vi "AIM664 Loopback.vi"() -> ()   [LabVIEW 2020]
uses:
  typedefs/BoardControlControl.ctl
  typedefs/BoardControlPortConfig.ctl
  typedefs/BoardControlGoodLink.ctl
  src/AIM664LV.lvlib
panel:
  out "QueueIdOut":u32 format="%x"
  out "GlobMonSize":u32 format="%x"
  in  "Strobe":u32(ring) items=["FDX_MON_STROBE_DIS", "FDX_MON_STROBE_STOP", "FDX_MON_STROBE_START"]
  in  "TriggerPosition":u32
  in  "CaptureMode":u32(ring) items=["FDX_MON_SINGLE ", "FDX_MON_CONTINUOUS", "FDX_MON_SELECTIVE", "FDX_MON_RECORDING", "FDX_MON_REROS", "FDX_MON_HMU"]
  out "Goodlink":bool
  out "error out":errorcluster
  in  "TxControl":T1={"StartMode"=1, "Count"=0, "Sign"=0, "Day"=0, "Hour"=0, "Min"=0, "Second"=0, "MilliSec"=0, "MicroSec"=0, "ExtendedStopMode"=0, "TransmitTime"=0} {"ExtendedStopMode" items=["FDX_ESTOP_NOT_USED", "FDX_ESTOP_EXT_TRG", "FDX_ESTOP_EXT_TRG_RESTART", "FDX_ESTOP_TIME"]; "StartMode" items=["FDX_STOP", "FDX_START", "FDX_START_TRG", "FDX_START_TIME"]}
  out "TxStatus":T2 {"TransmitMode" items=["FDX_TX_GENERIC", "FDX_TX_REPLAY", "FDX_TX_INDIVIDUAL"]; "TxStatus" items=["FDX_STAT_STOP", "FDX_STAT_RUN", "FDX_STAT_ERROR", "FDX_STAT_WAIT_F_TRIG"]}
  in  "TxQueueWriteIn":T3={"HeaderType"=0, "EntryCount"=1, "WriteBytes"=150, "FrameSize"=64, "FrameType"=0, "InterFrameGap"=1000, "PacketGroupWaitTime"=0, "PayloadBufferMode"=0, "PayloadGenerationMode"=0, "BufferQueueHandle"=0, "ExternalStrobe"=0, "PreambleCount"=0, "Skew"=1, "NetSelect"=0, "FrameStartMode"=0, "PhysErrorInjection"=0, "SequenceNumberInit"=65535, "SequenceNumberOffset"=65535, "Code"=0, "Interrupt"=0, "Data"=[3, 0, 0, 0, 0, 0, 2, 0, 0, 1, 1, 32, 8, 0, 69, 0, 0, 45, 0, 0, 64, 0, 1, 17, 141, 223, 10, 1, 1, 0, 224, 224, 0, 0, 0, 1, 0, 2, 0, 25, 0, 0, 65, 66, 67, 68, 69, 70, 71, 72, 73, 74, 75, 76, 77, 78, 79, 80, 81, 11]} {"Data" format="%x"; "FrameType" items=["FDX_TX_FRAME_STD", "FDX_TX_FRAME_INSTR"]; "SequenceNumberOffset" items=["FDX_TX_FRAME_SEQ_OFFS_AUTO "=65535]; "SequenceNumberInit" items=["FDX_TX_FRAME_SEQ_INIT_AUTO"=65535]; "PhysErrorInjection" items=["FDX_TX_FRAME_ERR_OFF"=0, "FDX_TX_FRAME_ERR_CRC"=1, "FDX_TX_FRAME_ERR_ALI"=2, "FDX_TX_FRAME_ERR_PRE"=4, "FDX_TX_FRAME_ERR_PHY"=8]; "FrameStartMode" items=["FDX_TX_FRAME_START_IFG", "FDX_TX_FRAME_START_PGWT", "FDX_TX_FRAME_START_TRG"]; "NetSelect" items=["FDX_TX_FRAME_DLY_A"=0, "FDX_TX_FRAME_DLY_B"=1, "FDX_TX_FRAME_BOTH "=3, "FDX_TX_FRAME_ONLY_A"=4, "FDX_TX_FRAME_ONLY_B "=5]; "PreambleCount" max=15; "ExternalStrobe" items=["FDX_DIS", "FDX_ENA"]; "PayloadGenerationMode" items=["FDX_TX_FRAME_PGM_USER"=0, "FDX_TX_FRAME_PGM_IP_PART"=1, "FDX_TX_FRAME_PGM_IP_FULL"=2, "FDX_TX_FRAME_PGM_IP_PART_TT"=10, "FDX_TX_FRAME_PGM_IP_FULL_TT"=20]; "PayloadBufferMode" items=["FDX_TX_FRAME_PBM_STD", "FDX_TX_FRAME_PBM_MAC", "FDX_TX_FRAME_PBM_UDP"]; "HeaderType" items=["FDX_TX_FRAME_HEADER_GENERIC ", "FDX_TX_FRAME_HEADER_REPLAY"]}
  out "ResourceInfo 2":T4 {"PortStructId" format="%x"; "PortMode" items=[" FDX_SINGLE", "FDX_REDUNDANT"]; "BoardStructId" format="%x"; "BoardShared\nMemSize" format="%x"; "BoardGlobal\nMemSize" format="%x"}
  out "ResourceInfo":T4 {"PortStructId" format="%x"; "PortMode" items=[" FDX_SINGLE", "FDX_REDUNDANT"]; "BoardStructId" format="%x"; "BoardShared\nMemSize" format="%x"; "BoardGlobal\nMemSize" format="%x"}
  out "Output Cluster 3":T6={"PortConfig"=[0, 0, 4294967295, 4294967295], "PortSpeed"=[0, 0, 4294967295, 4294967295], "PortUsed"=[1, 1, 0, 0], "PortGoodLink"=[1, 1, 4294967295, 4294967295], "ExpertMode"=[0, 0, 4294967295, 4294967295], "GlobalMemFree"=0, "SharedMemFree"=0, "RxVeriMode"=0} {"SharedMemFree" format="%x"; "GlobalMemFree" format="%x"; "ExpertMode" items=["FDX_EXPERT_MODE", "FDX_DISA_GHOST"]; "PortGoodLink" items=["FDX_NO_LINK", "FDX_GOOD_LINK"]; "PortSpeed" items=["FDX_100MBIT", "FDX_10MBIT", "FDX_AUTO_100MBIT", "FDX_AUTO_10MBIT"]; "PortConfig" items=["FDX_SINGLE", "FDX_REDUNDANT"]}
  in  "Input Cluster 3":T9={"Control"=1, "Port1ConfigIn"=0, "Port2ConfigIn"=0, "Port3ConfigIn"=0, "Port4ConfigIn"=0, "Port1SpeedIn"=0, "Port2SpeedIn"=0, "Port3SpeedIn"=0, "Port4SpeedIn"=0, "Expert1Mode"=0, "Expert2Mode"=0, "Expert3Mode"=0, "Expert4Mode"=0, "RxVeriModeIn"=0, "RxVeriData1"=0, "RxVeriData2"=0, "RxVeriData3"=0, "RxVeriData4"=0, "RxVeriData5"=0, "RxVeriData6"=0, "RxVeriData7"=0, "RxVerData8"=0, "RxVeriMask1"=0, "RxVeriMask2"=0, "RxVeriMask3"=0, "RxVeriMask4"=0, "RxVeriMask5"=0, "RxVeriMask6"=0, "RxVeriMask7"=0, "RxVeriMask8"=0} {"Expert4Mode" items=["FDX_EXPERT_MODE", "FDX_DISA_GHOST"]; "Expert3Mode" items=["FDX_EXPERT_MODE", "FDX_DISA_GHOST"]; "Expert2Mode" items=["FDX_EXPERT_MODE", "FDX_DISA_GHOST"]; "Expert1Mode" items=["FDX_EXPERT_MODE", "FDX_DISA_GHOST"]; "Port4SpeedIn" items=["FDX_100MBIT", "FDX_10MBIT", "FDX_AUTO_100MBIT", "FDX_AUTO_10MBIT"]; "Port3SpeedIn" items=["FDX_100MBIT", "FDX_10MBIT", "FDX_AUTO_100MBIT", "FDX_AUTO_10MBIT"]; "Port2SpeedIn" items=["FDX_100MBIT", "FDX_10MBIT", "FDX_AUTO_100MBIT", "FDX_AUTO_10MBIT"]; "Port1SpeedIn" items=["FDX_100MBIT", "FDX_10MBIT", "FDX_AUTO_100MBIT", "FDX_AUTO_10MBIT"]; "Port4ConfigIn" items=["FDX_SINGLE", "FDX_REDUNDANT"]; "Port3ConfigIn" items=["FDX_SINGLE", "FDX_REDUNDANT"]; "Port2ConfigIn" items=["FDX_SINGLE", "FDX_REDUNDANT"]; "Port1ConfigIn" items=["FDX_SINGLE", "FDX_REDUNDANT"]; "Control" items=["FDX_READ", "FDX_WRITE"]}
  out "Output Cluster":T10={"EntryRead"=0, "BytesRead"=0, "Synchronized"=0, "ReadBuffer"=[192, 121, 24, 2, 64, 122, 24, 2, 0, 0, 4, 4, 1, 0, 0, 0, 0, 0, 0, 0, 64, 64, 0, 80, 0, 0, 128, 0, 209, 8, 0, 0, 137, 2, 191, 69, 3, 0, 0, 0, 0, 0, 2, 0, 0, 1, 1, 32, 8, 0, 69, 0, 0, 45, 0, 0, 64, 0, 1, 17, 141, 223, 10, 1, 1, 0, 224, 224, 0, 0, 0, 1, 0, 2, 0, 25, 0, 0, 0, 0, 0, 0, 0, 0, 0, 0, 0, 0, 0, 0, 77, 78, 79, 80, 81, 0, 121, 63, 127, 127, 255, 254, 250, 252, 255, 251, 255, 255, 255, 223, 255, 255, 223, 255, 255, 255, 223, 255, 95, 223, 127, 127, 253, 55, 255, 251, 207, 253, 192, 121, 24, 2, 192, 122, 24, 2, 0, 0, 4, 0, 1, 0, 0, 0, 0, 0, 0, 0, 64, 0, 250, 64, 1, 0, 128, 0, 209, 8, 0, 0, 183, 2, 191, 69, 3, 0, 0, 0, 0, 0, 2, 0, 0, 1, 1, 32, 8, 0, 69, 0, 0, 45, 0, 0, 64, 0, 1, 17, 141, 223, 10, 1, 1, 0, 224, 224, 0, 0, 0, 1, 0, 2, 0, 25, 0, 0, 65, 66, 67, 68, 69, 70, 71, 72, 73, 74, 75, 76, 77, 78, 79, 80, 81, 1, 255, 123, 59, 123, 254, 222, 254, 255, 255, 247, 127, 247, 255, 239, 255, 253, 247, 191, 127, 255, 255, 222, 109, 253, 223, 255, 214, 251, 207, 222, 222, 206, 64, 122, 24, 2, 64, 123, 24, 2, 0, 0, 4, 0, 1, 0, 0, 0, 0, 0, 0, 0, 64, 0, 250, 64, 2, 0, 128, 0, 209, 8, 0, 0, 229, 2, 191, 69, 3, 0, 0, 0, 0, 0, 2, 0, 0, 1, 1, 32, 8, 0, 69, 0, 0, 45, 0, 0, 64, 0, 1, 17, 141, 223, 10, 1, 1, 0, 224, 224, 0, 0, 0, 1, 0, 2, 0, 25, 0, 0, 65, 66, 67, 68, 69, 70, 71, 72, 73, 74, 75, 76, 77, 78, 79, 80, 81, 2, 255, 255, 127, 127, 255, 255, 255, 223, 119, 239, 127, 123, 255, 207, 254, 253, 191, 123, 127, 127, 255, 223, 255, 222, 247, 127, 255, 251, 255, 255, 239, 255, 192, 122, 24, 2, 192, 123, 24, 2, 0, 0, 4, 0, 1, 0, 0, 0, 0, 0, 0, 0, 64, 0, 250, 64, 3, 0, 128, 0, 209, 8, 0, 0, 18, 3, 191, 69, 3, 0, 0, 0, 0, 0, 2, 0, 0, 1, 1, 32, 8, 0, 69, 0, 0, 45, 0, 0, 64, 0, 1, 17, 141, 223, 10, 1, 1, 0, 224, 224, 0, 0, 0, 1, 0, 2, 0, 25, 0, 0, 65, 66, 67, 68, 69, 70, 71, 72, 73, 74, 75, 76, 77, 78, 79, 80, 81, 3, 255, 250, 191, 255, 239, 255, 207, 222, 223, 251, 251, 63, 255, 237, 158, 215, 191, 127, 255, 255, 255, 254, 253, 255, 255, 127, 115, 251, 251, 254, 223, 94, 64, 123, 24, 2, 64, 124, 24, 2, 0, 0, 4, 0, 1, 0, 0, 0, 0, 0, 0, 0, 64, 0, 250, 64, 4, 0, 128, 0, 209, 8, 0, 0, 64, 3, 191, 69, 3, 0, 0, 0, 0, 0, 2, 0, 0, 1, 1, 32, 8, 0, 69, 0, 0, 45, 0, 0, 64, 0, 1, 17, 141, 223, 10, 1, 1, 0, 224, 224, 0, 0, 0, 1, 0, 2, 0, 25, 0, 0, 65, 66, 67, 68, 69, 70, 71, 72, 73, 74, 75, 76, 77, 78, 79, 80, 81, 4, 127, 255, 119, 127, 207, 239, 254, 95, 63, 127, 247, 23, 207, 211, 110, 250, 220, 255, 255, 187, 255, 223, 255, 254, 127, 247, 127, 187, 253, 238, 255, 223, 0, 0, 0, 0, 0, 0, 0, 0, 0, 0, 0, 0, 0, 0, 0, 0, 0, 0, 0, 0, 0, 0, 0, 0, 0, 0, 0, 0, 0, 0, 0, 0, 0, 0, 0, 0, 0, 0, 0, 0, 0, 0, 0, 0, 0, 0, 0, 0, 0, 0, 0, 0, 0, 0, 0, 0, 0, 0, 0, 0, 0, 0, 0, 0, 0, 0, 0, 0, 0, 0, 0, 0, 0, 0, 0, 0, 0, 0, 0, 0, 0, 0, 0, 0, 0, 0, 0, 0, 0, 0, 0, 0, 0, 0, 0, 0, 0, 0, 0, 0, 0, 0, 0, 0, 0, 0, 0, 0, 0, 0, 0, 0, 0, 0, 0, 0, 0, 0, 0, 0, 0, 0, 0, 0, 0, 0, 0, 0, 0, 0, 0, 0, 0, 0, 0, 0, 0, 0, 0, 0, 0, 0, 0, 0, 0, 0, 0, 0, 0, 0, 0, 0, 0, 0, 0, 0, 0, 0, 0, 0, 0, 0, 0, 0, 0, 0, 0, 0, 0, 0, 0, 0, 0, 0, 0, 0, 0, 0, 0, 0, 0, 0, 0, 0, 0, 0, 0, 0, 0, 0, 0, 0, 0, 0, 0, 0, 0, 0, 0, 0, 0, 0, 0, 0, 0, 0, 0, 0, 0, 0, 0, 0, 0, 0, 0, 0, 0, 0, 0, 0, 0, 0, 0, 0, 0, 0, 0, 0, 0, 0, 0, 0, 0, 0, 0, 0, 0, 0, 0, 0, 0, 0, 0, 0, 0, 0, 0, 0, 0, 0, 0, 0, 0, 0, 0, 0, 0, 0, 0, 0, 0, 0, 0, 0, 0, 0, 0, 0, 0, 0, 0, 0, 0, 0, 0, 0, 0, 0, 0, 0, 0, 0, 0, 0, 0, 0, 0, 0, 0, 0, 0, 0, 0, 0, 0, 0, 0, 0, 0, 0, 0, 0, 0, 0, 0, 0, 0, 0, 0, 0, 0, 0, 0, 0, 0, 0, 0, 0, 0, 0, 0, 0, 0, 0, 0, 0, 0, 0, 0, 0, 0, 0, 0, 0, 0, 0, 0, 0, 0, 0, 0, 0, 0, 0, 0, 0, 0, 0, 0, 0, 0, 0, 0, 0, 0, 0, 0, 0, 0, 0]} {"ReadBuffer" format="%x"}
  in  "Input Cluster":T11={"QueueId"=0, "EntryCount"=5, "ReadQualifier"=0, "MaxReadBytes"=1000} {"ReadQualifier" items=["FDX_MON_READ_FULL", "FDX_MON_READ_HEADER", "FDX_MON_READ_DATA"]}
  out "Output Cluster":T12={"TotalByteCount"=[0, 0, 0, 0, 0, 0, 0, 0], "FrameGoodCount"=[0, 0, 0, 0, 0, 0, 0, 0], "FrameErrorCount"=[0, 0, 0, 0, 0, 0, 0, 0], "BytesPerSecond"=[0, 0, 0, 0, 0, 0, 0, 0], "FramesPerSecond"=[0, 0, 0, 0, 0, 0, 0, 0], "PhysErrorCount"=[0, 0, 0, 0, 0, 0, 0, 0], "PreamErrorCount"=[0, 0, 0, 0, 0, 0, 0, 0], "UnaligErrorCount"=[0, 0, 0, 0, 0, 0, 0, 0], "CRCErrorCount"=[0, 0, 0, 0, 0, 0, 0, 0], "IFGErrorCount"=[0, 0, 0, 0, 0, 0, 0, 0], "IPErrorCount"=[0, 0, 0, 0, 0, 0, 0, 0], "MACErrorCount"=[0, 0, 0, 0, 0, 0, 0, 0], "NoSfdErrorCount"=[0, 0, 0, 0, 0, 0, 0, 0], "VLLenErrorCount"=[0, 0, 0, 0, 0, 0, 0, 0], "SNIntegrityErrorCount"=[0, 0, 0, 0, 0, 0, 0, 0], "TrafShapingViolationCount"=[0, 0, 0, 0, 0, 0, 0, 0], "MAC1Short"=[0, 0, 0, 0, 0, 0, 0, 0], "MAC64To127Count"=[100, 0, 0, 0, 0, 0, 0, 0], "MAC128To255Count"=[0, 0, 0, 0, 0, 0, 0, 0], "MAC256To511Count"=[0, 0, 0, 0, 0, 0, 0, 0], "MAC512To1023Count"=[0, 0, 0, 0, 0, 0, 0, 0], "MAC1024To1518Count"=[0, 0, 0, 0, 0, 0, 0, 0], "MACLong"=[0, 0, 0, 0, 0, 0, 0, 0]}
  in  "Control":u32(ring)=1 items=["FDX_RX_GS_RES_NO_CNT", "FDX_RX_GS_RES_ALL_CNT", "FDX_RX_GS_RES_ERR_CNT"]
  in  "Input Cluster":T1={"StartMode"=1, "Count"=100, "Sign"=0, "Day"=0, "Hour"=0, "Min"=0, "Second"=0, "MilliSec"=0, "MicroSec"=0, "ExtendedStopMode"=0, "TransmitTime"=0} {"ExtendedStopMode" items=["FDX_ESTOP_NOT_USED", "FDX_ESTOP_EXT_TRG", "FDX_ESTOP_EXT_TRG_RESTART", "FDX_ESTOP_TIME"]; "StartMode" items=["FDX_STOP", "FDX_START", "FDX_START_TRG", "FDX_START_TIME"]}
  out "Output Cluster":T13 {"MonStatus" items=["FDX_MON_OFF", "FDX_MON_WAIT_FOR_TRIGGER", "FDX_MON_TRIGGERED", "FDX_MON_STOPPED", "FDX_MON_FULL"]}
  in  "Input Cluster":T14 {"QueueCtrl" items=["FDX_MON_QUEUE_CREATE", "FDX_MON_QUEUE_DELETE"]}
  in  "Input Cluster":T15={"ReceiveMode"=0, "DefaultPayloadMode"=0, "DefaultCronoMode"=1, "GlbMonBufferSizeIn"=0, "RerosDefaultOutputPortmap"=0} {"DefaultCronoMode" items=["cFDX_RX_DEFAULT_ENA_CNT", "FDX_RX_DEFAULT_MON_ENA_ALL", "FDX_RX_DEFAULT_MON_ENA_GOOD"]; "DefaultPayloadMode" items=["FDX_PAYLOAD_FULL", "FDX_PAYLOAD_IP_EXT", "FDX_PAYLOAD_IP", "FDX_PAYLOAD_MAC"]; "ReceiveMode" items=["FDX_RX_CHRONO", "FDX_RX_VL"]}
  out "GlbMonBufferSizeOut":u32 format="%x"
  in  "Input Cluster":T16={"SrvName"="local", "ClHostName"="local", "ClUser"="Brett", "ClApplication"="Test", "ClApplicationVersion"="V01.00", "ResourceID"=3, "Privileges"=4294967295} {"Privileges" items=["PRIVILEGES_ADMIN"=4294967295]}
  out "Output Cluste":cluster{"QueueBaseAddr":u32, "QueueSizeOut":u32} {"QueueSizeOut" format="%x"; "QueueBaseAddr" format="%x"}
  in  "QueueSizeIn":u32
  in  "Input Cluster":T16={"SrvName"="local", "ClHostName"="local", "ClUser"="Brett", "ClApplication"="Test", "ClApplicationVersion"="V01.00", "ResourceID"=1, "Privileges"=4294967295} {"Privileges" items=["PRIVILEGES_ADMIN"=4294967295]}
  in  "Input Cluster":T17={"SrvName"="local", "ResourceID"=1, "ResourceType"=0} {"ResourceType" items=["Board", "Port"]}
  out "Output Cluster 2":T18={"ResourceID"=1, "ResourceType"=0, "ResourceInfo"="AMC-FDX-2", "StructId"=0}
  in  "ServerRElement":u32=1
  in  "PortMap":u32
  out "Output Cluster":T19={"PortConfig"=0, "PortUsed"=1, "GlobalMemFree"=0, "SharedMemFree"=0} {"SharedMemFree" format="%x"; "GlobalMemFree" format="%x"; "PortConfig" items=["FDX_SINGLE", "FDX_REDUNDANT"]}
  in  "RerosPortDelay":u32
  in  "TransmitMode":u32(ring) items=["FDX_TX_GENERIC", "FDX_TX_REPLAY", "FDX_TX_INDIVIDUAL"]
  in  "Input Cluster":T17={"SrvName"="local", "ResourceID"=2, "ResourceType"=1} {"ResourceType" items=["Board", "Port"]}
  in  "Input Cluster":T16={"SrvName"="local", "ClHostName"="local", "ClUser"="Brett", "ClApplication"="Test", "ClApplicationVersion"="V01.00", "ResourceID"=2, "Privileges"=4294967295} {"Privileges" items=["PRIVILEGES_ADMIN"=4294967295]}
  out "Output Cluster":T18={"ResourceID"=2, "ResourceType"=1, "ResourceInfo"="Port1", "StructId"=0}
  in  "ServerRElement":u32=2
  out "NuOfResources":u32=3
  in  "SrvName":string="local"
  out "NuOfServers":u32=1
  # "ARINC 664 Loopback"
  # "Overview: Performs a Loopback between Port 1 and Port 2 of the board.\nRequirement: One AIM ARINC-664 board with installed AIM ARINC 664 BSP.\nRestrictions: none.\nInstruction:\n1. Connect a Port 1 to Port 2 of the board\n2. Run the VI.\n3. If no error happen, you have estabished connection between both ports."
  # "Rx Port"
  # "Tx Port"
  # "Board"
  # "Tx Port"
  # "Rx Port"
  # "Board"
  # "FdxRxControlCvi"
  # "FdxInitCvi"
  # "FdxLogoutCvi"
  # "CountServerResourcesCvi"
  # "GetServerResourcesCvi"
  # "QueryServerResourceCvi"
  # "FdxLoginCvi"
  # "FdxLoginCvi"
  # "FdxBoardControlCvi"
  # "FdxLogoutCvi"
  # "FdxLogoutCvi"
  # "GetServerResourcesCvi"
  # "QueryServerResourceCvi"
  # "FdxTxModeControlCvi"
  # "FdxTxQueueCreateCvi"
  # "FdxTxQueueWriteCvi"
  # "FdxTxControlCvi"
  # "FdxTxStatusCvi"
  # "FdxTxControlCvi"
  # "FdxRxModeControlCvi"
  # "FdxRxMonCaptureControlCvi"
  # "FdxCmdRxGlobalStatisticsCvii"
  # "FdxLoginCvi"
  # "FdxCmdMonQueueControl"
  # "FdxRxControlCvi"
  # "FdxMonGetStatusCvii"
  # "FdxCmdMonQueueReadCvii"
  # "FdxTxPortInitCvi"
  # "Input"
  # "Input"
  # "Input"
  # "Input"
  # "Input"
  # "Input"
  # "Input"
  # "Input"
  # "Input"
  # "Input"
  # "Input"
  # "Input"
  # "Input"
  # "Input"
  # "Input"
  # "Output"
  # "Input"
  # "Input"
  # "Input"
  # "Input"
  # "Input"
  # "Input"
  # "Input"
  # "Input"
  # "Input"
  # "Input"
  # "Input"
  # "Output"
  # "Output"
  # "Output"
  # "Output"
  # "Output"
  # "Output"
  # "Output"
  # "Output"
  # "Output"
  # "Output"
  # "Output"
  # "Output"
  # "Output"
  # "Output"
  # "Output"
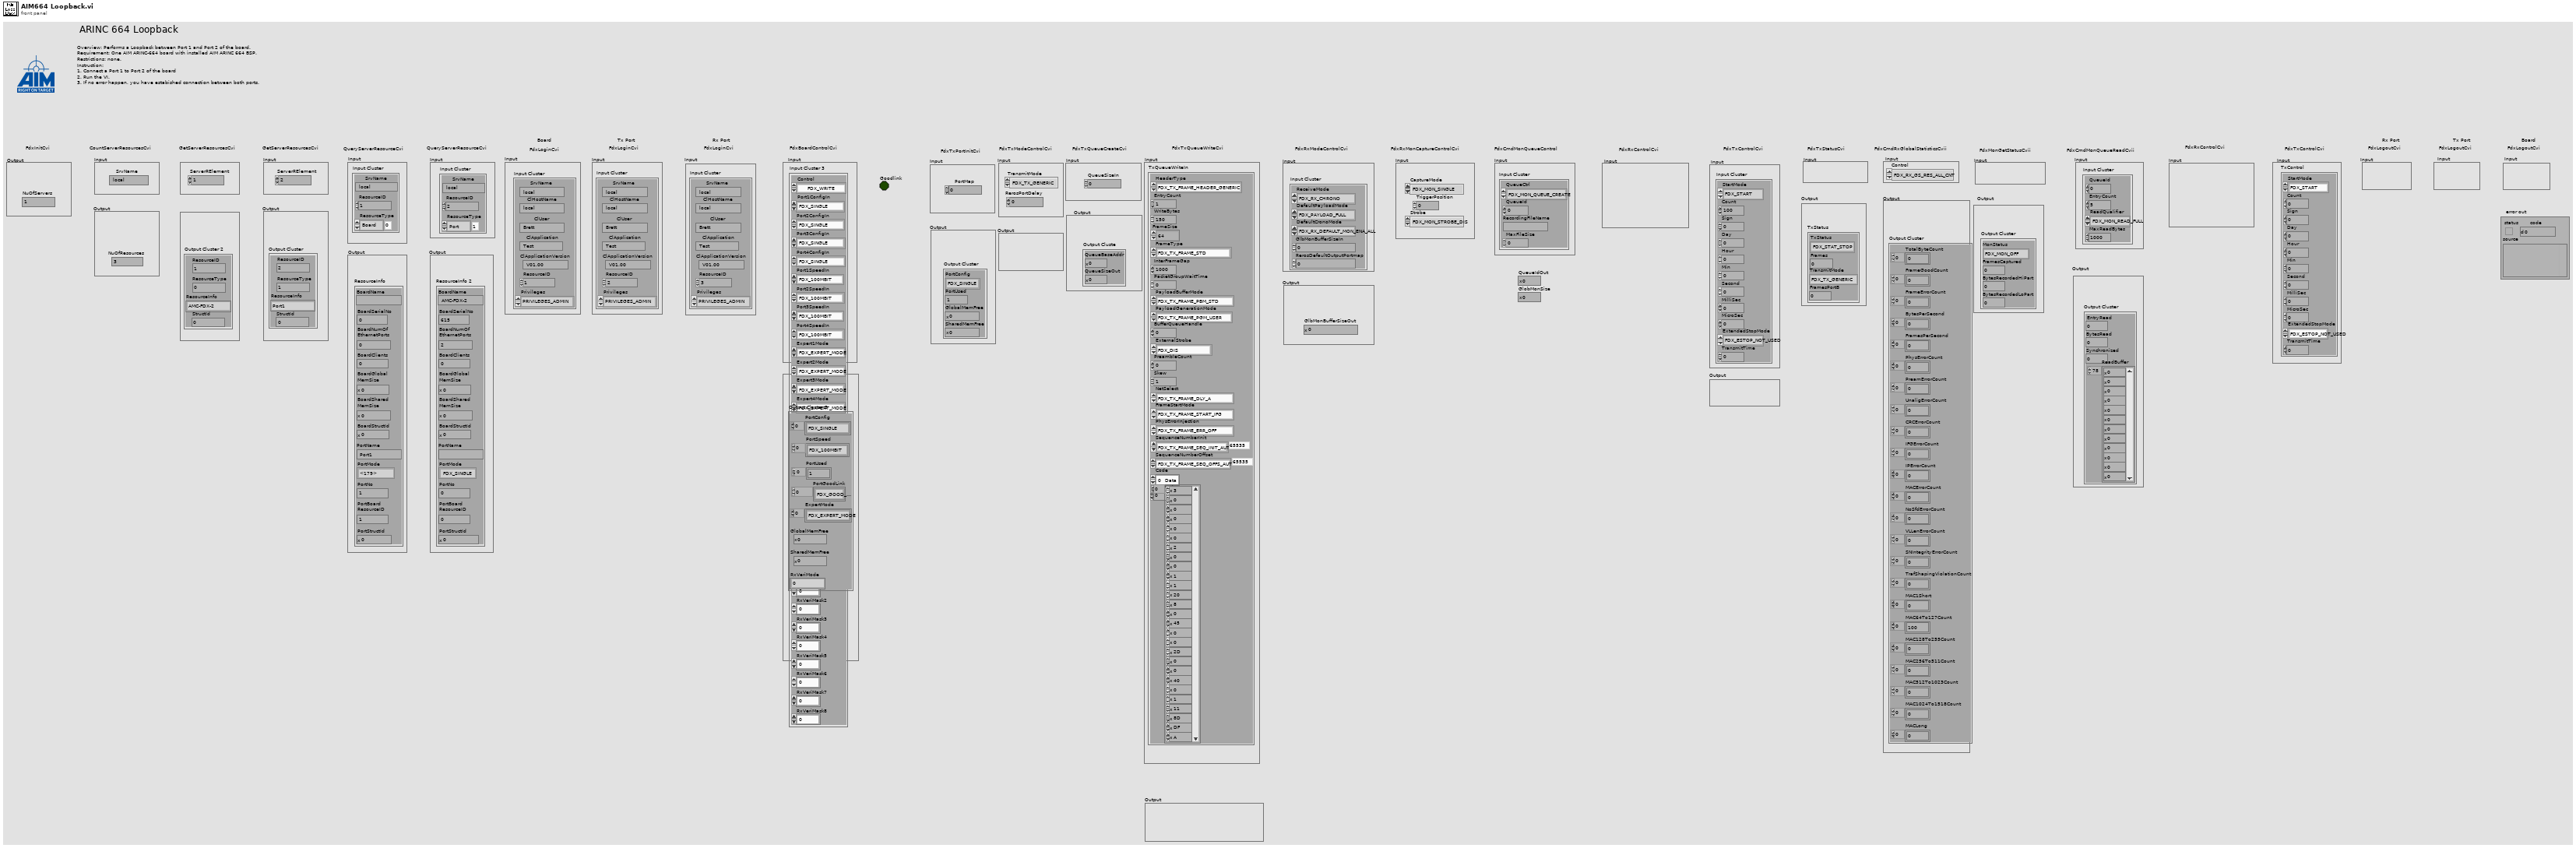
[diagram p1: front panel]
types:
  T1 = cluster{"StartMode":i32, "Count":u32, "Sign":i32, "Day":u32, "Hour":u32, "Min":u32, "Second":u32, "MilliSec":u32, "MicroSec":u32, "ExtendedStopMode":i32, "TransmitTime":u32}
  T2 = cluster{"TxStatus":u32, "Frames":u32, "TransmitMode":u32, "FramesPortB":u32}
  T3 = cluster{"HeaderType":u32, "EntryCount":u32, "WriteBytes":u32, "FrameSize":u16, "FrameType":u8, "InterFrameGap":u32, "PacketGroupWaitTime":u32, "PayloadBufferMode":u8, "PayloadGenerationMode":u8, "BufferQueueHandle":u32, "ExternalStrobe":u8, "PreambleCount":u8, "Skew":u32, "NetSelect":u8, "FrameStartMode":u8, "PhysErrorInjection":u32, "SequenceNumberInit":u16, "SequenceNumberOffset":u16, "Code":u8, "Interrupt":u8, "Data":u8[]}
  T4 = cluster{"BoardName":string, "BoardSerialNo":u32, "BoardNumOf\nEthernetPorts":u32, "BoardClients":u32, "BoardGlobal\nMemSize":u32, "BoardShared\nMemSize":u32, "BoardStructId":u32, "PortName":string, "PortMode":u32, "PortNo":u32, "PortBoard\nResourceID":u32, "PortStructId":u32}
  T5 = typedef "BoardControlGoodLink.ctl" = u32
  T6 = cluster{"PortConfig":u32[], "PortSpeed":u32[], "PortUsed":u32[], "PortGoodLink":T5[], "ExpertMode":u32[], "GlobalMemFree":u32, "SharedMemFree":u32, "RxVeriMode":u32}
  T7 = typedef "BoardControlControl.ctl" = u32
  T8 = typedef "BoardControlPortConfig.ctl" = u32
  T9 = cluster{"Control":T7, "Port1ConfigIn":T8, "Port2ConfigIn":u32, "Port3ConfigIn":u32, "Port4ConfigIn":i32, "Port1SpeedIn":u32, "Port2SpeedIn":u32, "Port3SpeedIn":u32, "Port4SpeedIn":u32, "Expert1Mode":u32, "Expert2Mode":u32, "Expert3Mode":u32, "Expert4Mode":u32, "RxVeriModeIn":u32, "RxVeriData1":u32, "RxVeriData2":u32, "RxVeriData3":u32, "RxVeriData4":u32, "RxVeriData5":u32, "RxVeriData6":u32, "RxVeriData7":u32, "RxVerData8":u32, "RxVeriMask1":u32, "RxVeriMask2":u32, "RxVeriMask3":u32, "RxVeriMask4":u32, "RxVeriMask5":u32, "RxVeriMask6":u32, "RxVeriMask7":u32, "RxVeriMask8":u32}
  T10 = cluster{"EntryRead":u32, "BytesRead":u32, "Synchronized":u32, "ReadBuffer":u8[]}
  T11 = cluster{"QueueId":u32, "EntryCount":u32, "ReadQualifier":u32, "MaxReadBytes":u32}
  T12 = cluster{"TotalByteCount":u32[], "FrameGoodCount":u32[], "FrameErrorCount":u32[], "BytesPerSecond":u32[], "FramesPerSecond":u32[], "PhysErrorCount":u32[], "PreamErrorCount":u32[], "UnaligErrorCount":u32[], "CRCErrorCount":u32[], "IFGErrorCount":u32[], "IPErrorCount":u32[], "MACErrorCount":u32[], "NoSfdErrorCount":u32[], "VLLenErrorCount":u32[], "SNIntegrityErrorCount":u32[], "TrafShapingViolationCount":u32[], "MAC1Short":u32[], "MAC64To127Count":u32[], "MAC128To255Count":u32[], "MAC256To511Count":u32[], "MAC512To1023Count":u32[], "MAC1024To1518Count":u32[], "MACLong":u32[]}
  T13 = cluster{"MonStatus":u32, "FramesCaptured":u32, "BytesRecordedHiPart":u32, "BytesRecordedLoPart":u32}
  T14 = cluster{"QueueCtrl":u32, "QueueId":u32, "RecordingFileName":string, "MaxFileSize":u32}
  T15 = cluster{"ReceiveMode":u32, "DefaultPayloadMode":u32, "DefaultCronoMode":u32, "GlbMonBufferSizeIn":u32, "RerosDefaultOutputPortmap":u32}
  T16 = cluster{"SrvName":string, "ClHostName":string, "ClUser":string, "ClApplication":string, "ClApplicationVersion":string, "ResourceID":u32, "Privileges":u32}
  T17 = cluster{"SrvName":string, "ResourceID":u32, "ResourceType":u32}
  T18 = cluster{"ResourceID":u32, "ResourceType":u32, "ResourceInfo":string, "StructId":u32}
  T19 = cluster{"PortConfig":u32, "PortUsed":u32, "GlobalMemFree":u32, "SharedMemFree":u32}
  T20 = typedef "AIM664LV.lvlib/port_configuration.ctl" = u32
  T21 = typedef "AIM664LV.lvlib/port_speed.ctl" = u32
  T22 = typedef "AIM664LV.lvlib/port_condition.ctl" = u32
  T23 = typedef "AIM664LV.lvlib/expert_mode.ctl" = u32
  T24 = cluster{"PortConfig":T20[], "PortSpeed":T21[], "PortUsed":u32[], "PortGoodLink":T22[], "ExpertMode":T23[], "GlobalMemFree":u32, "SharedMemFree":u32, "RxVeriMode":u32}
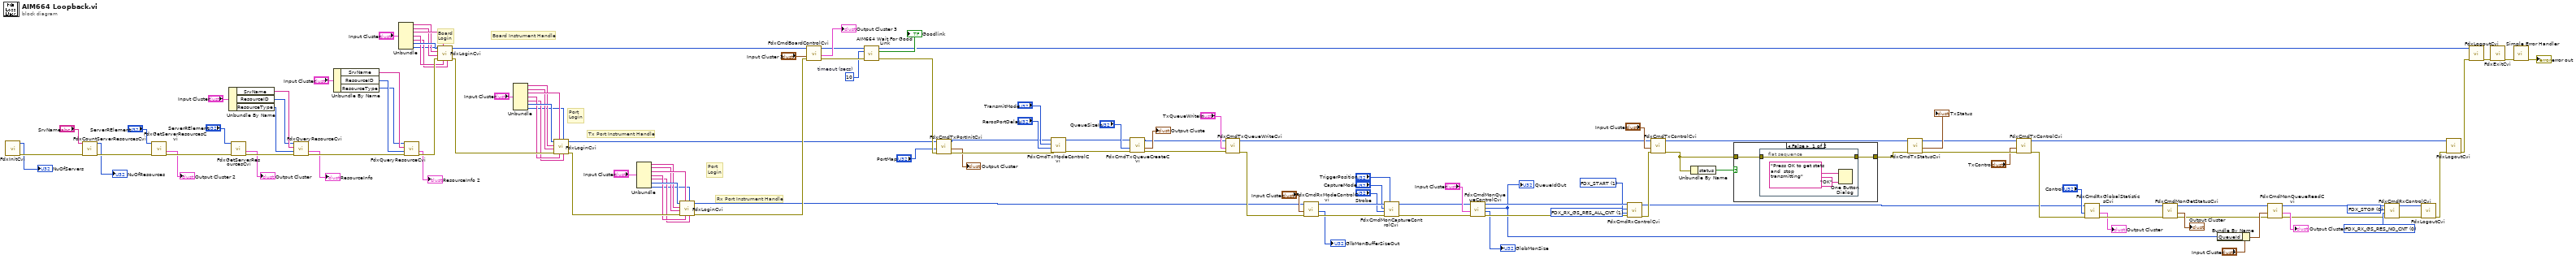
[diagram p0: block diagram]
diagram:
  w9 = u32 0 items=["FDX_RX_GS_RES_NO_CNT", "FDX_RX_GS_RES_ALL_CNT", "FDX_RX_GS_RES_ERR_CNT "] ("GlobalStatisticReset")
  w10 = u32 0 items=["FDX_STOP", "FDX_START"] ("StartMode")
  w11 = u32 1 items=["FDX_RX_GS_RES_NO_CNT", "FDX_RX_GS_RES_ALL_CNT", "FDX_RX_GS_RES_ERR_CNT "] ("GlobalStatisticReset")
  w12 = u32 1 items=["FDX_STOP", "FDX_START"] ("StartMode")
  w71 = 10  # timeout (secs)
  # "Rx Port Instrument Handle"
  # "Port\nLogin"
  # "Tx Port Instrument Handle"
  # "Board Instrument Handle"
  # "Port\nLogin"
  # "Board\nLogin"
  n1 = call "FdxInitCvi.vi"() -> ("error out"=w123:errorcluster, "Number of Servers"=→"NuOfServers":u32)  [unwired: 10 in]
  n2 = call "FdxCountServerResourcesCvi.vi"("error in"=w123, "SrvName (local)"="SrvName") -> ("error out"=w122:errorcluster, "Number of Resources"=→"NuOfResources":u32)  [unwired: 8 in]
  n3 = call "FdxGetServerResourcesCvi.vi"("error in"=w122, "ServerRElement"="ServerRElement") -> ("error out"=w121:errorcluster, "ServerResourceInfo"=→"Output Cluster 2":T18)  [unwired: 4 in, 4 out]
  n4 = Unbundle By Name("Input Cluster") -> ("SrvName"=w66:string, "ResourceID"=w64:u32, "ResourceType"=w63:u32)
  n5 = call "FdxGetServerResourcesCvi.vi"("error in"=w121, "ServerRElement"="ServerRElement") -> ("error out"=w126:errorcluster, "ServerResourceInfo"=→"Output Cluster":T18)  [unwired: 4 in, 4 out]
  n6 = call "FdxQueryResourceCvi.vi"("error in"=w126, "ResourceType"=w63, "SrvName"=w66, "ResourceID"=w64) -> ("error out"=w120:errorcluster, "ResourceInfo"=→"ResourceInfo":T4)  [unwired: 5 in, 1 out]
  n7 = Unbundle By Name("Input Cluster") -> ("SrvName"=w62:string, "ResourceID"=w61:u32, "ResourceType"=w60:u32)
  n8 = Unbundle("Input Cluster") -> ("SrvName"=w56:string, "ClHostName"=w55:string, "ClUser"=w57:string, "ClApplication"=w54:string, "ClApplicationVersion"=w53:string, "ResourceID"=w58:u32, "Privileges"=w52:u32)
  n9 = call "FdxQueryResourceCvi.vi"("error in"=w120, "ResourceType"=w61, "SrvName"=w62, "ResourceID"=w60) -> ("error out"=w119:errorcluster, "ResourceInfo"=→"ResourceInfo 2":T4)  [unwired: 5 in, 1 out]
  n10 = call "FdxLoginCvi.vi"("ClApplicationVersion"=w53, "Privileges"=w52, "ClApplication"=w54, "ClUser"=w57, "error in"=w119, "ClHostName"=w55, "SrvName"=w56, "ResourceID"=w58) -> ("error out"=w101:errorcluster, "InstrumentHandle"=w73:u32)  [unwired: 2 in]
  n11 = Unbundle("Input Cluster") -> ("SrvName"=w49:string, "ClHostName"=w48:string, "ClUser"=w50:string, "ClApplication"=w47:string, "ClApplicationVersion"=w46:string, "ResourceID"=w51:u32, "Privileges"=w45:u32)
  n12 = call "FdxLoginCvi.vi"("ClApplicationVersion"=w46, "Privileges"=w45, "ClApplication"=w47, "ClUser"=w50, "error in"=w101, "ClHostName"=w48, "SrvName"=w49, "ResourceID"=w51) -> ("error out"=w100:errorcluster, "InstrumentHandle"=w43:u32)  [unwired: 2 in]
  n13 = Unbundle("Input Cluster") -> ("SrvName"=w40:string, "ClHostName"=w39:string, "ClUser"=w41:string, "ClApplication"=w38:string, "ClApplicationVersion"=w37:string, "ResourceID"=w42:u32, "Privileges"=w36:u32)
  n14 = call "FdxLoginCvi.vi"("ClApplicationVersion"=w37, "Privileges"=w36, "ClApplication"=w38, "ClUser"=w41, "error in"=w100, "ClHostName"=w39, "SrvName"=w40, "ResourceID"=w42) -> ("error out"=w99:errorcluster, "InstrumentHandle"=w35:u32)  [unwired: 2 in]
  n15 = call "FdxCmdBoardControlCvi.vi"("error in"=w99, "BoardControlIn (read)"="Input Cluster 3", "InstrumentHandle_board in"=w73) -> ("error out"=w104:errorcluster, "Board Control Out"=→"Output Cluster 3":T24, "InstrumentHandle_board out"=w25:u32)  [unwired: 6 in]
  n16 = call "AIM664 Wait For Good Link.vi"("error in"=w104, "timeout (secs)"=w71, "InstrumentHandle_board in"=w25) -> ("error out"=w103:errorcluster, "Goodlink"=→"Goodlink":bool, "InstrumentHandle_board out"=w24:u32)  [unwired: 6 in]
  n17 = call "FdxCmdTxPortInitCvi.vi"("error in"=w103, "PortMap"="PortMap", "InstrumentHandle_port"=w43) -> ("error out"=w125:errorcluster, "PortInitOut"=→"Output Cluster":T19, "InstrumentHandle_port"=w33:u32)  [unwired: 6 in]
  n18 = call "FdxCmdTxModeControlCvi.vi"("error in"=w125, "RerosPortDelay"="RerosPortDelay", "TransmitMode"="TransmitMode", "InstrumentHandle_port"=w33) -> ("error out"=w118:errorcluster, "InstrumentHandle_port"=w32:u32)  [unwired: 6 in]
  n19 = call "FdxCmdTxQueueCreateCvi.vi"("error in"=w118, "QueueSizeIn"="QueueSizeIn", "InstrumentHandle_port"=w32) -> ("error out"=w117:errorcluster, "TxQueueInfo"=→"Output Cluste":cluster{"QueueBaseAddr":u32, "QueueSizeOut":u32}, "InstrumentHandle_port"=w31:u32)  [unwired: 6 in]
  n20 = call "FdxCmdTxQueueWriteCvi.vi"("error in"=w117, "TxQueueWriteIn"="TxQueueWriteIn", "InstrumentHandle_port"=w31) -> ("error out"=w109:errorcluster, "InstrumentHandle_port"=w30:u32)  [unwired: 7 in]
  n21 = call "FdxCmdRxModeControlCvi.vi"("error in"=w109, "RxModeControlIn"="Input Cluster", "InstrumentHandle_port"=w35) -> ("error out"=w113:errorcluster, "GlbMonBufferSizeOut"=→"GlbMonBufferSizeOut":u32, "InstrumentHandle_port"=w23:u32)  [unwired: 6 in]
  n22 = call "FdxCmdMonCaptureControlCvi.vi"("TriggerPosition"="TriggerPosition", "error in"=w113, "Strobe"="Strobe", "CaptureMode"="CaptureMode", "InstrumentHandle_port"=w23) -> ("error out"=w112:errorcluster, "InstrumentHandle_port"=w22:u32)  [unwired: 5 in]
  n23 = call "FdxCmdMonQueueControlCvi.vi"("error in"=w112, "Q Ctrl In"="Input Cluster", "InstrumentHandle_port"=w22) -> ("error out"=w111:errorcluster, "GlobMonSize"=→"GlobMonSize":u32, "QueueIdOut"=w14:u32, "InstrumentHandle_port"=w21:u32)  [unwired: 5 in]
  "QueueIdOut" <- w14
  n24 = call "FdxCmdRxControlCvi.vi"("error in"=w111, "GlobalStatisticReset"=w11, "StartMode"=w12, "InstrumentHandle_port"=w21) -> ("error out"=w110:errorcluster, "InstrumentHandle_port"=w20:u32)  [unwired: 6 in]
  n25 = call "FdxCmdTxControlCvi.vi"("error in"=w110, "TxControl"="Input Cluster", "InstrumentHandle_port"=w30) -> ("error out"=w102:errorcluster, "InstrumentHandle_port"=w29:u32)  [unwired: 7 in]
  n26 = Unbundle By Name(w102) -> ("status"=w72:bool)
  n27 = case shown="False" w72 {
    tunnel: w102 -> [w128 w132]
    tunnel: [w127 w132] -> w124
    frame False {
      n28 = flat-sequence {
        tunnel: w128 -> [w131]
        tunnel: [w131] -> w127
        frame #0 {
          n29 = One Button Dialog(message="Press OK to get stats and  stop transmitting", button name ("OK")="OK") -> ()  [unwired: 1 out]
        }
      }
    }
    frame True {
    }
  }
  n30 = call "FdxCmdTxStatusCvi.vi"("error in"=w124, "InstrumentHandle_port"=w29) -> ("error out"=w116:errorcluster, "TxStatus"=→"TxStatus":T2, "InstrumentHandle_port"=w28:u32)  [unwired: 7 in]
  n31 = call "FdxCmdTxControlCvi.vi"("error in"=w116, "TxControl"="TxControl", "InstrumentHandle_port"=w28) -> ("error out"=w107:errorcluster, "InstrumentHandle_port"=w27:u32)  [unwired: 7 in]
  n32 = call "FdxCmdRxGlobalStatisticsCvi.vi"("error in"=w107, "Control"="Control", "InstrumentHandle_port"=w20) -> ("error out"=w106:errorcluster, "GlobalStat Out"=→"Output Cluster":T12, "InstrumentHandle_port"=w19:u32)  [unwired: 6 in]
  n33 = call "FdxCmdMonGetStatusCvi.vi"("error in"=w106, "InstrumentHandle_port"=w19) -> ("error out"=w6:errorcluster, "MonStatus"=→"Output Cluster":T13, "InstrumentHandle_port"=w7:u32)  [unwired: 7 in]
  n34 = Bundle By Name(cluster="Input Cluster", "QueueId"=w14) -> (w8:T11)
  n35 = call "FdxCmdMonQueueReadCvi.vi"("error in"=w6, "QueueReadIn"=w8, "InstrumentHandle_port"=w7) -> ("error out"=w4:errorcluster, "QueueReadOut"=→"Output Cluster":T10, "InstrumentHandle_port"=w3:u32)  [unwired: 6 in]
  n36 = call "FdxCmdRxControlCvi.vi"("error in"=w4, "GlobalStatisticReset"=w9, "StartMode"=w10, "InstrumentHandle_port"=w3) -> ("error out"=w108:errorcluster, "InstrumentHandle_port"=w18:u32)  [unwired: 6 in]
  n37 = call "FdxLogoutCvi.vi"("error in"=w108, "InstrumentHandle"=w18) -> ("error out"=w115:errorcluster)  [unwired: 9 in]
  n38 = call "FdxLogoutCvi.vi"("error in"=w115, "InstrumentHandle"=w27) -> ("error out"=w114:errorcluster)  [unwired: 9 in]
  n39 = call "FdxLogoutCvi.vi"("error in"=w114, "InstrumentHandle"=w24) -> ("error out"=w105:errorcluster)  [unwired: 9 in]
  n40 = call "FdxExitCvi.vi"("error in"=w105) -> ("error out"=w2:errorcluster)  [unwired: 10 in]
  n41 = call <vilib>:"Simple Error Handler.vi"("error in (no error)"=w2) -> ("error out"=→"error out":errorcluster)  [unwired: 4 in, 4 out]
